vi "PADMINI_STATUS_COLOR_CHANGE .vi"(10 "Numeric":u16, 11 "Boolean in":refnum<vi>) -> ()   [LabVIEW 2017]
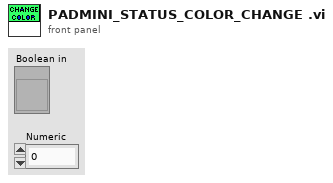
[diagram p1: front panel]
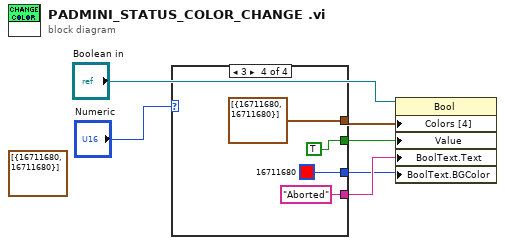
[diagram p0: block diagram]
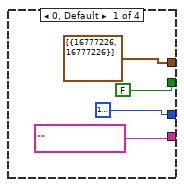
[diagram p2: hidden frame]
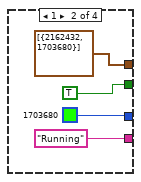
[diagram p3: hidden frame]
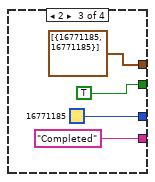
[diagram p4: hidden frame]
diagram:
  (unwired) cluster{u32, u32}[] [{16711680, 16711680}] ("Colors [4]")
  n1 = case shown="3" "Numeric" {
    tunnel: [cluster{u32, u32}[] [{16777226, 16777226}] ("Colors [4]") cluster{u32, u32}[] [{2162432, 1703680}] ("Colors [4]") cluster{u32, u32}[] [{16771185, 16771185}] ("Colors [4]") cluster{u32, u32}[] [{16711680, 16711680}] ("Colors [4]")] -> w3
    tunnel: [FALSE TRUE TRUE TRUE] -> w4
    tunnel: ["" "Running" "Completed" "Aborted"] -> w2
    tunnel: [u32 16777226 u32 1703680 u32 16771185 u32 16711680] -> w1
    frame 0, Default {
    }
    frame 1 {
    }
    frame 2 {
    }
    frame 3 {
    }
  }
  n2 = property on="Property Node" class="Bool"(reference="Boolean in", "Colors [4]"=w3, "Value"=w4, "BoolText.Text"=w2, "BoolText.BGColor"=w1) -> ()  [unwired: 1 in, 2 out]
